vi "testGetRange.vi"() -> ()   [LabVIEW 2016]
uses:
  Electrometer/Electrometer.lvclass
  ElectrometerConfiguration/ElectrometerConfiguration.lvclass
panel:
  out "Range":string
  in  "VISA":refnum<visa-resource-name>
  out "error out":errorcluster
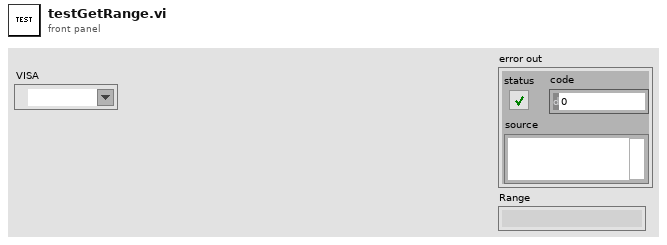
[diagram p1: front panel]
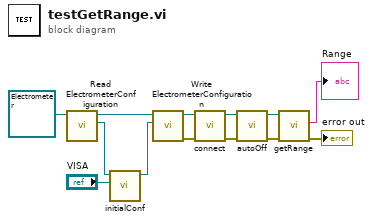
[diagram p0: block diagram]
diagram:
  n1 = call-dynamic "Read ElectrometerConfiguration.vi"("Electrometer in"=refnum<class "Electrometer.lvclass"> refnum ("Electrometer.lvclass")) -> ("ElectrometerConfiguration"=w11:refnum<class "ElectrometerConfiguration.lvclass">, "Electrometer out"=w12:refnum<class "Electrometer.lvclass">)  [unwired: 8 in, 1 out]
  n2 = call "initialConf.vi"("VISA"="VISA", "ElectrometerConfiguration In"=w11) -> ("ElectrometerConfiguration Out"=w10:refnum<class "ElectrometerConfiguration.lvclass">)  [unwired: 9 in]
  n3 = call-dynamic "Write ElectrometerConfiguration.vi"("ElectrometerConfiguration"=w10, "Electrometer in"=w12) -> ("error out"=w8:errorcluster, "Electrometer out"=w9:refnum<class "Electrometer.lvclass">)  [unwired: 8 in]
  n4 = call "connect.vi"("error in (no error)"=w8, "Electrometer in"=w9) -> ("error out"=w6:errorcluster, "Electrometer out"=w7:refnum<class "Electrometer.lvclass">)  [unwired: 7 in, 1 out]
  n5 = call "autoOff.vi"("error in (no error)"=w6, "Electrometer in"=w7) -> ("error out"=w3:errorcluster, "Electrometer out"=w4:refnum<class "Electrometer.lvclass">)  [unwired: 8 in]
  n6 = call "getRange.vi"("error in (no error)"=w3, "Electrometer in"=w4) -> ("error out"=→"error out":errorcluster, "Range"=→"Range":string)  [unwired: 7 in, 1 out]
